vi "Update.vi"(9 "Column":i32, 10 "Row":i32, 11 "64 in":refnum<class "Picture.lvclass">) -> (3 "64 out":refnum<class "Picture.lvclass">)   [LabVIEW 2015, in "Picture.lvclass"]
uses:
  Picture.lvclass
  64 Type.ctl
  Common/Position.ctl
  Picture.lvclass/Picture.ctl
  SubVIs/Read-Only Globals.vi
  SubVIs/Globals (private).vi
  Square/Square.lvclass
  Common/Common.lvlib
panel:
  out "Locations":i32[][](array[numeric])
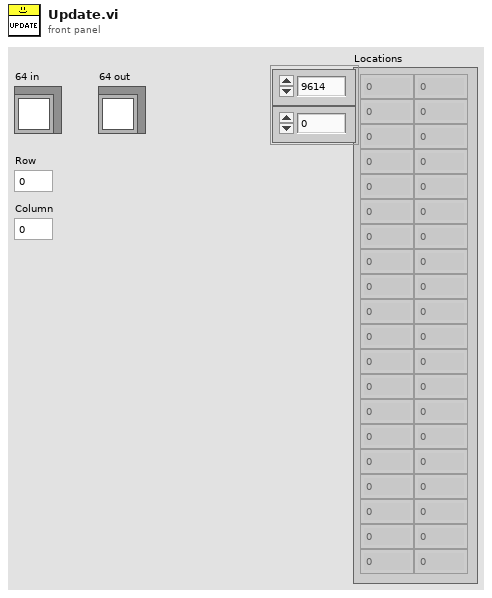
[diagram p1: front panel]
types:
  T1 = typedef "Picture.lvclass/64 Type.ctl" = enum16{"Starter", "Expander"}
  T2 = typedef "Common.lvlib/Position.ctl" = cluster{"Column":i32, "Row":i32}
  T3 = typedef "Common.lvlib/Map DVR.ctl" = refnum<data-value>
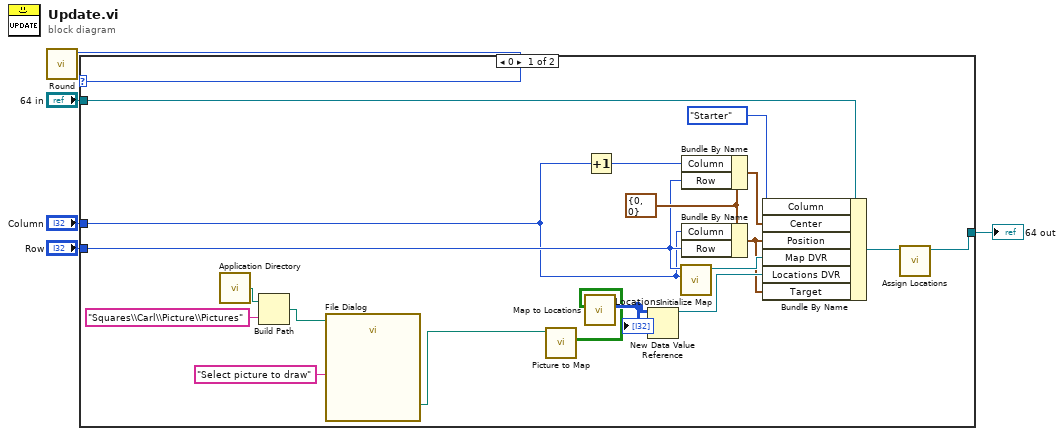
[diagram p0: block diagram]
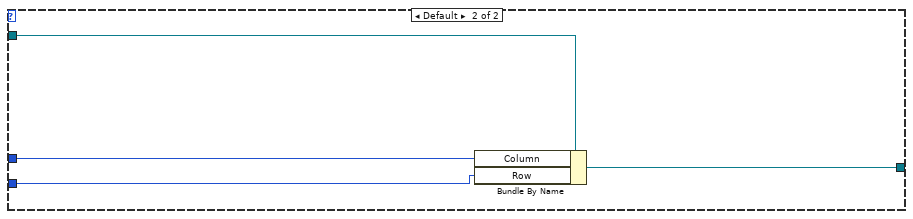
[diagram p2: hidden frame]
diagram:
  n1 = call "Round.vi"() -> ("Round"=w3:i32)  [unwired: 11 in]
  n2 = case shown="0" w3 {
    tunnel: "64 in" -> [w24 w28]
    tunnel: [w12 w27] -> w4
    tunnel: "Row" -> [w17 w25]
    tunnel: "Column" -> [w16 w26]
    frame 0 {
      w19 = T2 {"Column"=0, "Row"=0} ("Center")
      n3 = call <vilib>:"Application Directory.vi"() -> ("Application Directory"=w8:path)
      n4 = Build Path(base path=w8, name or relative path="Squares\\Carl\\Picture\\Pictures") -> (appended path=w6:path)
      n5 = call "File Dialog"("start path"=w6, "prompt"="Select picture to draw") -> ("selected path"=w9:path)  [unwired: 10 in, 3 out]
      n6 = call "Picture to Map.vi"("path to JPEG file"=w9) -> ("Map out"=w11:bool[][])  [unwired: 10 in]
      n7 = call "Map to Locations.vi"("Map in"=w11) -> ("Locations"=w14:i32[][])  [unwired: 10 in]
      "Locations" <- w14
      n8 = Increment(x=w16) -> (x+1=w21:i32)
      n9 = New Data Value Reference(data value=w14) -> (data value reference=w15:refnum<data-value>)  [unwired: 1 in, 1 out]
      n10 = call "Initialize Map.vi"("Column"=w16, "Row"=w17) -> ("Map DVR"=w18:T3)  [unwired: 9 in]
      n11 = Bundle By Name(cluster=w19, "Column"=w21, "Row"=w17) -> (w20:T2)
      n12 = Bundle By Name(cluster=w19, "Column"=w16, "Row"=w17) -> (w13:T2)
      n13 = Bundle By Name(cluster=w24, "Column"=64_Type."Starter" ("Type"), "Center"=w20, "Position"=w13, "Map DVR"=w18, "Locations DVR"=w15, "Target"=w13) -> (w23:refnum<class "Picture.lvclass">)
      n14 = call "Assign Locations.vi"("Picture In"=w23) -> ("Picture Out"=w12:refnum<class "Picture.lvclass">)  [unwired: 9 in, 1 out]
    }
    frame Default {
      n15 = Bundle By Name(cluster=w28, "Column"=w26, "Row"=w25) -> (w27:refnum<class "Picture.lvclass">)
    }
  }
  "64 out" <- w4
